vi "FormatVersionString.vi"(0 "Version":T1, 1 "delimiter":string=".", 2 "mark revision":bool) -> (3 "Version string":string)   [LabVIEW 2014, in "RasPiDownloader.lvlib"]
uses:
  RasPiDownloader.lvlib
  RuntimeVersion.ctl
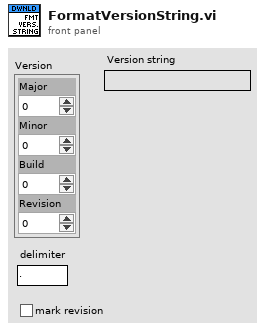
[diagram p1: front panel]
types:
  T1 = typedef "RasPiDownloader.lvlib/RuntimeVersion.ctl" = cluster{"Major":i32, "Minor":i32, "Build":i32, "Revision":i32}
  T2 = cluster{"Major":string, "Minor":string, "Build":string, "Revision":string}
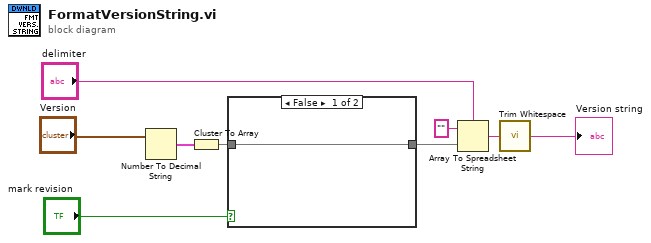
[diagram p0: block diagram]
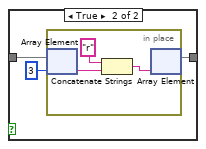
[diagram p2: hidden frame]
diagram:
  n1 = Number To Decimal String(number="Version") -> (decimal integer string=w8:T2)  [unwired: 1 in]
  n2 = Cluster To Array(cluster=w8) -> (array=w2:string[])
  n3 = case shown="False" "mark revision" {
    tunnel: w2 -> [w10 w13]
    tunnel: [w10 w11] -> w1
    frame False {
    }
    frame True {
      n4 = in-place {
        n5 = in-place-array #1(w13, 3) -> (w16:string)
        n6 = Concatenate Strings("r" ("string"), w16) -> (w15:string)
        n7 = in-place-array #1(w15) -> (w11:string[])  [unwired: 1 out]
      }
    }
  }
  n8 = Array To Spreadsheet String(delimiter (Tab)="delimiter", array=w1, 3:"" ("format string")) -> (spreadsheet string=w5:string)
  n9 = call <vilib>:"Trim Whitespace.vi"("string"=w5) -> ("trimmed string"=→"Version string":string)  [unwired: 1 in]
